vi "Personality Version Results.vi"(0 "Expected Personality":string, 1 "Expected Version":string, 5 "Expected Model":string, 7 "ERD Data Out":T1[](array[typedef]) {"ERD Number" format="%.0x"}, 11 "Error In":errorcluster) -> (3 "Actual Personality":u8, 4 "Actual Model ID":u8, 6 "Boolean":bool, 8 "Report Text":string, 10 "Actual Version":string, 15 "Error Out":errorcluster)   [LabVIEW 2016]
uses:
  Common/LabVIEW GEA2 Toolkit/LabVIEW_GEA2_Toolkit.lvlibp/type defs/ERD Read Data Out.ctl
  Common/LabVIEW GEA2 Toolkit/LabVIEW_GEA2_Toolkit.lvlibp
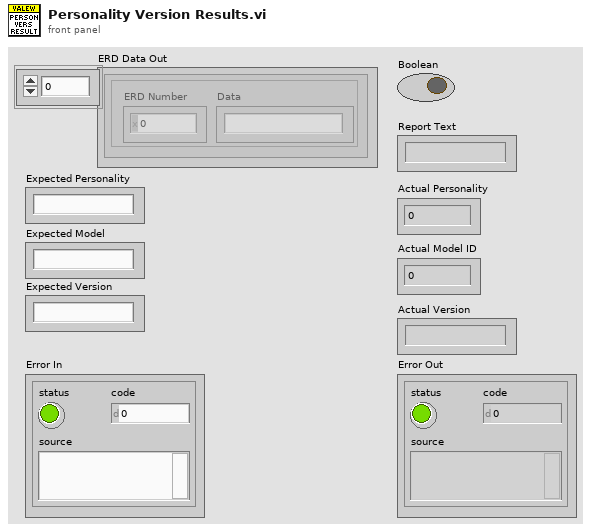
[diagram p1: front panel]
types:
  T1 = typedef "LabVIEW_GEA2_Toolkit.lvlibp/ERD Read Data Out.ctl" = cluster{"ERD Number":u16, "Data":string}
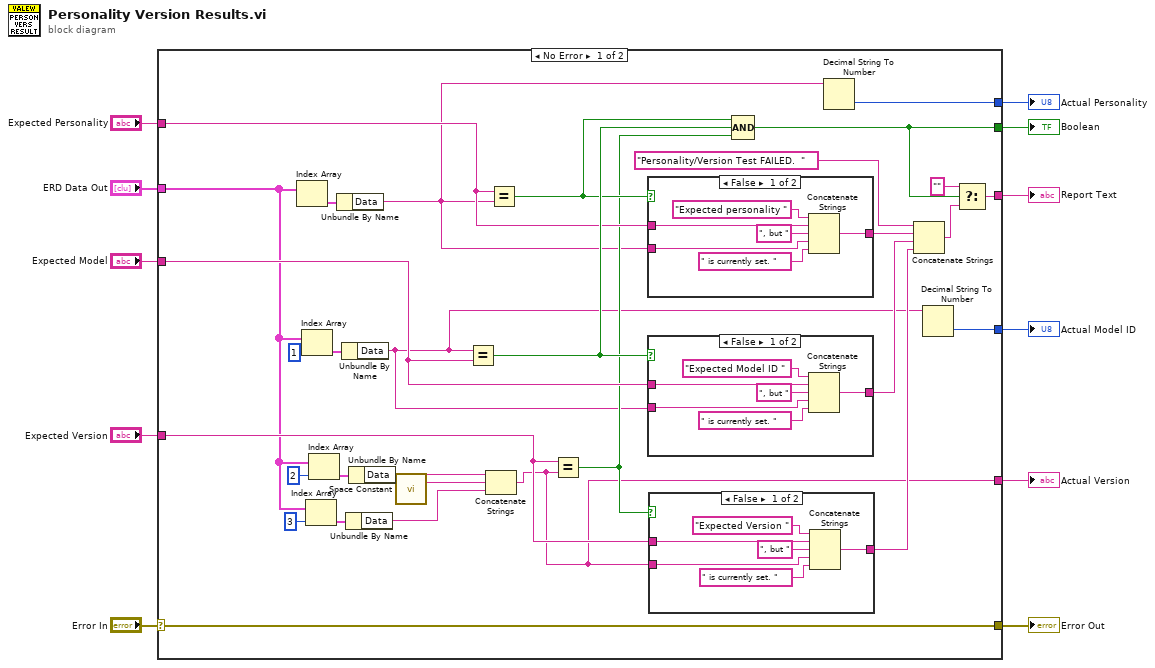
[diagram p0: block diagram]
diagram:
  n1 = case shown="No Error" "Error In" {
    selector: "Error In" -> [w25 w61]
    tunnel: [w42 _] -> w11
    tunnel: "Expected Model" -> [w36 _]
    tunnel: "Expected Personality" -> [w33 _]
    tunnel: [w32 _] -> w8
    tunnel: [w25 w61] -> w6
    tunnel: "Expected Version" -> [w20 _]
    tunnel: "ERD Data Out" -> [w18 _]
    tunnel: [w16 _] -> w3
    tunnel: [w14 _] -> w2
    tunnel: [w13 _] -> w1
    frame No Error {
      n2 = Index Array(array=w18) -> (element=w30:T1)  [unwired: 1 in]
      n3 = Index Array(array=w18, index=1) -> (element=w34:T1)
      n4 = Index Array(array=w18, index=3) -> (element=w29:T1)
      n5 = Index Array(array=w18, index=2) -> (element=w26:T1)
      n6 = Unbundle By Name(w30) -> ("Data"=w17:string)
      n7 = Unbundle By Name(w34) -> ("Data"=w15:string)
      n8 = Unbundle By Name(w29) -> ("Data"=w23:string)
      n9 = Unbundle By Name(w26) -> ("Data"=w24:string)
      n10 = call <vilib>:"Space Constant.vi"() -> ("String"=w22:string)
      n11 = Equal?(x=w15, y=w36) -> (x = y?=w41:bool)
      n12 = Concatenate Strings(w24, w22, w23) -> (w13:string)
      n13 = Equal?(x=w33, y=w17) -> (x = y?=w40:bool)
      n14 = Equal?(x=w20, y=w13) -> (x = y?=w19:bool)
      n15 = case shown="False" w40 {
        tunnel: [w59 _] -> w37
        tunnel: w33 -> [w58 _]
        tunnel: w17 -> [w56 _]
        frame False {
          n16 = Concatenate Strings("Expected personality " ("string"), w58, ", but " ("string"), w56, " is currently set. " ("string")) -> (w59:string)
        }
        frame True {
        }
      }
      n17 = case shown="False" w41 {
        tunnel: [w53 _] -> w38
        tunnel: w36 -> [w52 _]
        tunnel: w15 -> [w50 _]
        frame False {
          n18 = Concatenate Strings("Expected Model ID " ("string"), w52, ", but " ("string"), w50, " is currently set. " ("string")) -> (w53:string)
        }
        frame True {
        }
      }
      n19 = case shown="False" w19 {
        tunnel: [w47 _] -> w21
        tunnel: w20 -> [w46 _]
        tunnel: w13 -> [w44 _]
        frame False {
          n20 = Concatenate Strings("Expected Version " ("string"), w46, ", but " ("string"), w44, " is currently set. " ("string")) -> (w47:string)
        }
        frame True {
        }
      }
      n21 = Compound Arithmetic op=AND(w40, w41, w19) -> (w42:bool)
      n22 = Decimal String To Number(string=w17) -> (number=w16:i32)  [unwired: 2 in, 1 out]
      n23 = Concatenate Strings("Personality/Version Test FAILED.  " ("string"), w37, w38, w21) -> (w39:string)
      n24 = Decimal String To Number(string=w15) -> (number=w14:i32)  [unwired: 2 in, 1 out]
      n25 = Select(t="" ("Report Text"), s=w42, f=w39) -> (s? t:f=w32:string)
    }
    frame Error {
    }
  }
  "Boolean" <- w11
  "Report Text" <- w8
  "Error Out" <- w6
  "Actual Personality" <- w3
  "Actual Model ID" <- w2
  "Actual Version" <- w1
